vi "Read U32.vi"(8 "error in (no error)":errorcluster, 9 "Type":u32, 10 "Tag":string, 11 "Var Bus in":refnum<class "Omni_Bus.lvclass">) -> (0 "error out":errorcluster, 2 "Numeric":u32, 3 "Var Bus out":refnum<class "Omni_Bus.lvclass">)   [LabVIEW 2021, in "Omni_Bus.lvclass"]
uses:
  Omni_Bus.lvclass
  <vilib>/TSA/Abstract Data Classes/Abs_Types/U32 Integer/Abs_U32 Integer.lvclass
  Omni_Bus.lvclass/Omni_Bus.ctl
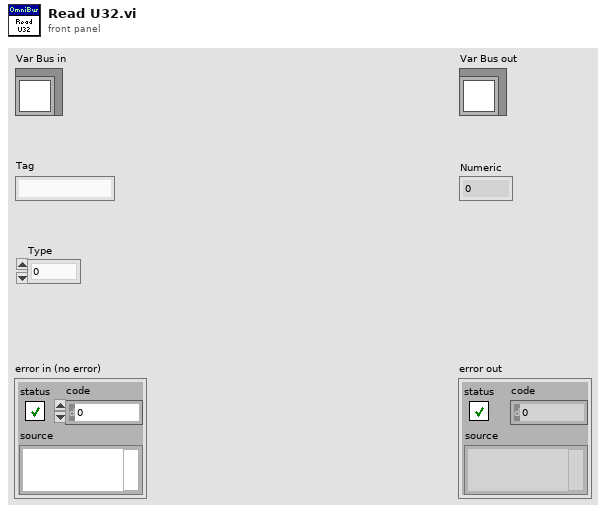
[diagram p1: front panel]
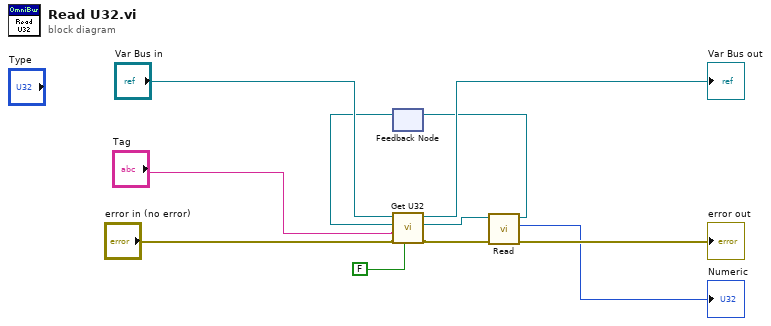
[diagram p0: block diagram]
diagram:
  n1 = feedback #1() -> (w2:refnum<class "Abs_U32 Integer.lvclass">)  [unwired: 1 in]
  n2 = call-dynamic "Get U32.vi"("Write?"=FALSE, "error in (no error)"="error in (no error)", "Tag"="Tag", "Value Type"=w2, "Var Bus in"="Var Bus in") -> ("error out"=w4:errorcluster, "Value Out"=w3:refnum<class "Abs_U32 Integer.lvclass">, "Var Bus out"=→"Var Bus out":refnum<class "Omni_Bus.lvclass">)  [unwired: 4 in]
  n3 = call-dynamic "Read.vi"("error in (no error)"=w4, "Double Float.lvclass_340760 in"=w3) -> ("error out"=→"error out":errorcluster, "Value"=→"Numeric":u32, "Double Float.lvclass_340760 out"=w5:refnum<class "Abs_U32 Integer.lvclass">)  [unwired: 7 in]
  n4 = feedback-in #1(w5) -> ()
